vi "Read Scores.vi"(6 "Start Time":timestamp, 11 "Score INI":path) -> (0 "error out":errorcluster, 1 "Error Code":i32, 2 "Test Summary":string, 3 "Score":T1)   [LabVIEW 2020, in "Summer of LabVIEW.lvlib" / "Scorer.lvclass"]
uses:
  Scorer.lvclass
  SoL Scoring/Score.ctl
  SoL Scoring/Score Entry.ctl
  <vilib>/Utility/config.llb/Read Key (I32).vi
  <vilib>/Utility/config.llb/Read Key (String).vi
  <vilib>/Utility/config.llb/Read Key (Double).vi
  <vilib>/Utility/config.llb/NI_LVConfig.lvlib
  SoL Scoring/SoL Scoring.lvlib
panel:
  out "Run Time":dbl format="%<%M:%S>t"
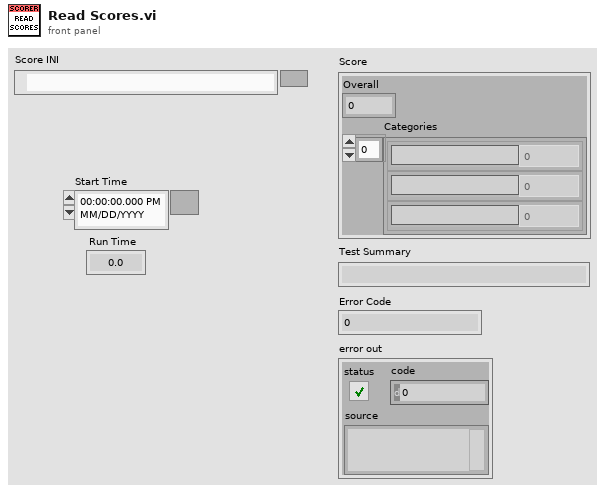
[diagram p1: front panel]
types:
  T1 = typedef "SoL Scoring.lvlib/Score.ctl" = cluster{"Overall":dbl, "Categories":T2[]}
  T2 = typedef "SoL Scoring.lvlib/Score Entry.ctl" = cluster{"Category":string, "Value":dbl}
  T3 = typedef "NI_LVConfig.lvlib/Config Data RefNum.ctl" = refnum<k1>
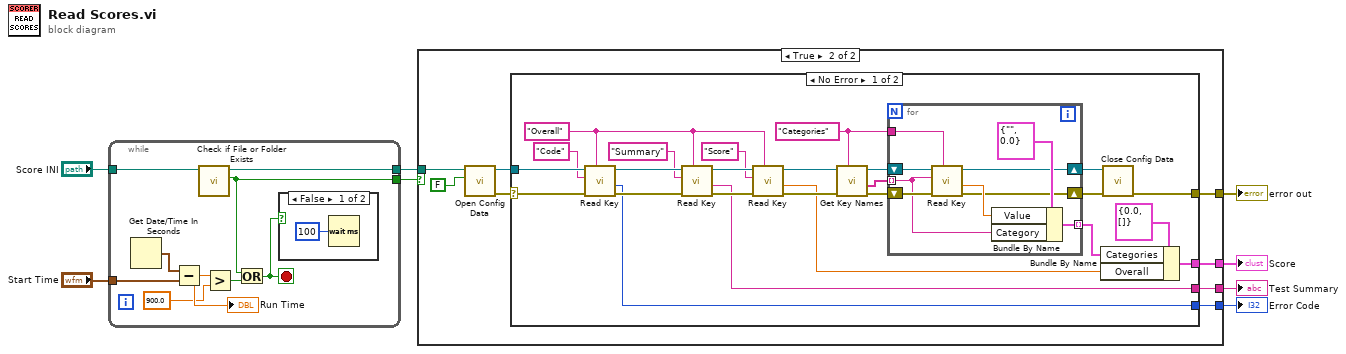
[diagram p0: block diagram]
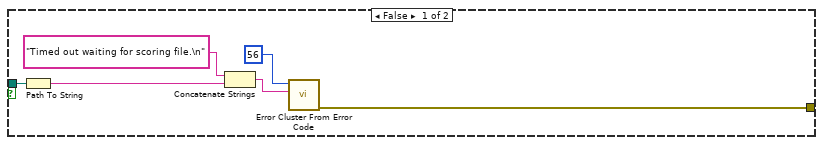
[diagram p2: hidden frame]
diagram:
  n1 = while {
    tunnel: "Start Time" -> [w17]
    tunnel: "Score INI" -> [w13]
    tunnel: [w11] -> w2
    tunnel: [w9] -> w1
    stop <- w10 stop-if-true
    n2 = Get Date/Time In Seconds() -> (seconds since 1Jan1904=w16:timestamp)
    n3 = Subtract(x=w16, y=w17) -> (x-y=w15:dbl)
    "Run Time" <- w15
    n4 = call <vilib>:"Check if File or Folder Exists.vi"("path"=w13) -> ("file or folder exists?"=w9:bool, "dup path"=w11:path)  [unwired: 8 in, 1 out]
    n5 = Greater?(x=w15, y=900.0) -> (0:w12:bool)
    n6 = Or(x=w9, y=w12) -> (x .or. y?=w10:bool)
    n7 = case shown="False" w10 {
      frame False {
        n8 = Wait (ms)(milliseconds to wait=u32 100) -> ()  [unwired: 1 out]
      }
      frame True {
      }
    }
  }
  n9 = case shown="True" w1 {
    tunnel: [w24 w29] -> w8
    tunnel: [_ w28] -> w7
    tunnel: [_ w27] -> w6
    tunnel: [_ w26] -> w5
    tunnel: w2 -> [w22 w25]
    frame False {
      n10 = Path To String(path=w22) -> (string=w21:string)
      n11 = Concatenate Strings("Timed out waiting for scoring file.\n", w21) -> (w19:string)
      n12 = call <vilib>:"Error Cluster From Error Code.vi"("error message (\"\")"=w19, "error code (0)"=56) -> ("error out"=w24:errorcluster)  [unwired: 7 in]
    }
    frame True {
      n13 = call <vilib>:"Open Config Data.vi"("create file if necessary (T)"=FALSE, "configuration file path"=w25) -> ("error out"=w30:errorcluster, "refnum"=w31:T3)  [unwired: 7 in, 1 out]
      n14 = case shown="No Error" w30 {
        selector: w30 -> [w55 w67]
        tunnel: w31 -> [w56 _]
        tunnel: [w39 w67] -> w29
        tunnel: [w35 _] -> w28
        tunnel: [w34 _] -> w27
        tunnel: [w33 _] -> w26
        frame No Error {
          w42 = "Categories" ("section")
          w48 = "Overall" ("section")
          n15 = call-poly <vilib>:"Read Key.vi"("section"=w48, "error in (no error)"=w55, "key"="Code", "refnum"=w56) -> ("error out"=w52:errorcluster, "value"=w34:i32, "refnum out"=w53:T3)  [unwired: 4 in, 1 out]
          n16 = call-poly <vilib>:"Read Key.vi"("section"=w48, "error in (no error)"=w52, "key"="Summary", "refnum"=w53) -> ("error out"=w49:errorcluster, "value"=w33:string, "refnum out"=w57:T3)  [unwired: 4 in, 1 out]
          n17 = call-poly <vilib>:"Read Key.vi"("section"=w48, "error in (no error)"=w49, "key"="Score", "refnum"=w57) -> ("error out"=w46:errorcluster, "value"=w36:dbl, "refnum out"=w47:T3)  [unwired: 4 in, 1 out]
          n18 = call <vilib>:"Get Key Names.vi"("section"=w42, "error in (no error)"=w46, "refnum"=w47) -> ("error out"=w44:errorcluster, "key names"=w43:string[], "refnum out"=w45:T3)  [unwired: 5 in, 1 out]
          n19 = for {
            shift-right: [w61] -> w41
            shift-left: w45 -> [w66]
            shift-right: [w60] -> w40
            shift-left: w44 -> [w65]
            tunnel: w43 -> [w58] mode=indexing
            tunnel: w42 -> [w64]
            tunnel: [w59] -> w37 mode=indexing
            n20 = call-poly <vilib>:"Read Key.vi"("section"=w64, "error in (no error)"=w65, "key"=w58, "refnum"=w66) -> ("error out"=w60:errorcluster, "value"=w62:dbl, "refnum out"=w61:T3)  [unwired: 4 in, 1 out]
            n21 = Bundle By Name(cluster=T2 {"Category"="", "Value"=0.0} ("Score Entry"), "Value"=w62, "Category"=w58) -> (w59:T2)
          }
          n22 = Bundle By Name(cluster=T1 {"Overall"=0.0, "Categories"=[]} ("Score"), "Categories"=w37, "Overall"=w36) -> (w35:T1)
          n23 = call <vilib>:"Close Config Data.vi"("error in (no error)"=w40, "refnum"=w41) -> ("error out"=w39:errorcluster)  [unwired: 8 in, 1 out]
        }
        frame Error {
        }
      }
    }
  }
  "Score" <- w7
  "Test Summary" <- w5
  "Error Code" <- w6
  "error out" <- w8
